vi "Save As Measurement Service template.vi"(8 "error in":errorcluster, 10 "measurement service name":string, 11 "project ref":refnum<vi>) -> (0 "error out":errorcluster, 3 "project ref out":refnum<vi>)   [LabVIEW 2021, in "MeasurementService Editor.lvlib"]
uses:
  MeasurementService Editor.lvlib
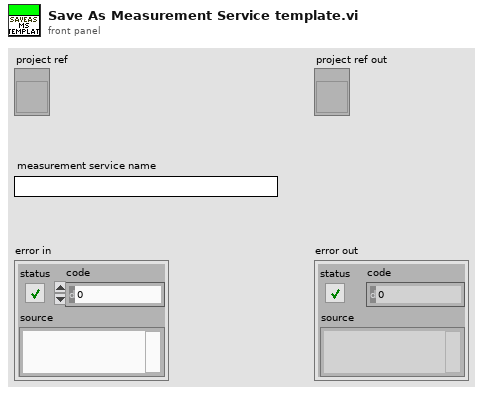
[diagram p1: front panel]
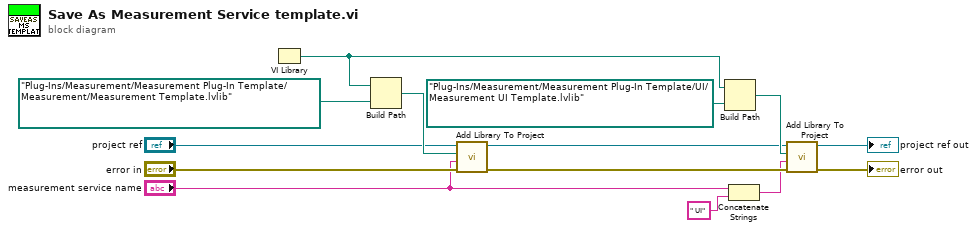
[diagram p0: block diagram]
diagram:
  n1 = VI Library() -> (path=w11:path)
  n2 = Build Path(base path=w11, name or relative path=path "Plug-Ins/Measurement/Measurement Plug-In Template/Measurement/Measurement Template.lvlib" ("Library Path")) -> (appended path=w13:path)
  n3 = call "Add Library To Project.vi"("error in"="error in", "new library name"="measurement service name", "library path"=w13, "project ref"="project ref") -> ("error out"=w12:errorcluster, "project ref out"=w2:refnum<vi>)  [unwired: 6 in]
  n4 = Build Path(base path=w11, name or relative path=path "Plug-Ins/Measurement/Measurement Plug-In Template/UI/Measurement UI Template.lvlib" ("Library Path")) -> (appended path=w10:path)
  n5 = Concatenate Strings("measurement service name", " UI" ("string")) -> (w9:string)
  n6 = call "Add Library To Project.vi"("error in"=w12, "new library name"=w9, "library path"=w10, "project ref"=w2) -> ("error out"=→"error out":errorcluster, "project ref out"=→"project ref out":refnum<vi>)  [unwired: 6 in]
